vi "GetExeVersion.vi"(11 "路径":path) -> (3 "Version of Executable":string)   [LabVIEW 2017]
panel:
  # "Cut and Paste code from the block diagram  \njust before you build the exectable. Remember \nthis code will give you an error if you try to run\n your program without building it into an executable."
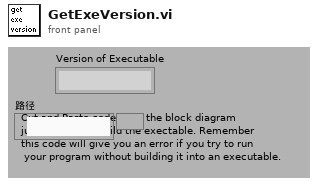
[diagram p1: front panel]
types:
  T1 = enum32{"invalid app kind", "Development System", "Run Time System", "Student Edition", "Embedded LabVIEW", "Evaluation", "Custom"}
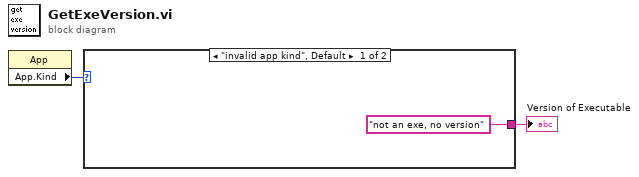
[diagram p0: block diagram]
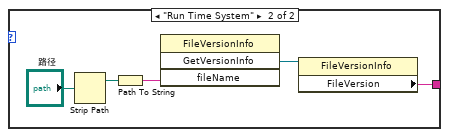
[diagram p2: hidden frame]
diagram:
  n1 = property class="App"() -> ("App.Kind"=w2:T1)  [unwired: 2 in, 2 out]
  n2 = case shown="\"invalid app kind\", Default" w2 {
    tunnel: ["not an exe, no version" ("FileVersion") w4] -> w1
    frame "invalid app kind", Default {
    }
    frame "Run Time System" {
      n3 = Strip Path(path="路径") -> (stripped path=w7:path)  [unwired: 1 out]
      n4 = Path To String(path=w7) -> (string=w5:string)
      n5 = invoke class="FileVersionInfo" method="GetVersionInfo"("fileName"=w5) -> ("GetVersionInfo"=w6:refnum<k24>)  [unwired: 3 in, 3 out]
      n6 = property class="FileVersionInfo"(reference=w6) -> ("FileVersion"=w4:string)  [unwired: 1 in, 2 out]
    }
  }
  "Version of Executable" <- w1
